vi "Fetch Measurement (More).vi"(0 "VISA resource name":refnum<visa-resource-name>, 5 "Measurement Source (1: Channel 1)":i32(ring)=1 caption="Channel (1: Channel 1)" items=["Channel 1"=1, "Channel 2"=2, "Channel 3"=3, "Channel 4"=4, "Function 1"=5, "Function 2"=6, "Function 3"=7, "Function 4"=8, "Memory 1"=9, "Memory 2"=10, "Memory 3"=11, "Memory 4"=12, "Clock"=15, "MTrend"=16, "MSpectrum"=17, "Equalized"=18, "DIG 0"=20, "DIG 1"=21, "DIG 2"=22, "DIG 3"=23, "DIG 4"=24, "DIG 5"=25, "DIG 6"=26, "DIG 7"=27, "DIG 8"=28, "DIG 9"=29, "DIG 10"=30, "DIG 11"=31, "DIG 12"=32, "DIG 13"=33, "DIG 14"=34, "DIG 15"=35], 7 "Measurement Function (0: Rise Time)":i32(ring) items=["Rise Time", "Fall Time", "Frequency", "Period", "Voltage RMS (AC)", "Voltage RMS (DC)", "Voltage RMS (AC,cycle)", "Voltage RMS (DC,cycle)", "Voltage Max", "Voltage Min", "Voltage Middle", "Voltage Vpp", "Voltage High", "Voltage Low", "Voltage Average", "Voltage Average (cycle)", "Width Negative", "Width Positive", "Duty Cycle Positive", "Amplitude", "Overshoot", "Preshoot", "Voltage Base", "Voltage Upper", "Time Max", "Time Min", "Color Grade Crossing", "Color Grade Eye Width", "Color Grade Eye Height", "Color Grade Eye Q-Factory", "Color Grade Eye Duty Cycle Distortion (Percent)", "Color Grade Eye Duty Cycle Distortion (Time)", "Color Grade Eye Jitter (PP)", "Color Grade Eye Width (RMS)", "Cycle-cycle Duty Jitter (Rising)", "Cycle-cycle Duty Jitter (Falling)", "Cycle-cycle Jitter (Rising)", "Cycle-cycle Jitter (Falling)", "Cycle-cycle - Width", "Cycle-cycle + Width", "Date Rate", "Unit Interval", "FFT Delta Frequency", "FFT Delta Magnitude", "FFT Frequency", "FFT Magnitude", "Slew Rate", "Area (Entire Display)", "Area (Single Cycle)", "Duty Cycle (Rising)", "Duty Cycle (Falling)", "Clock Recovery Rate", "Color Grade Eye Height (Measured)", "Color Grade Eye Height (Extrapolated)", "Color Grade Eye Width (Measured)", "Color Grade Eye width (Extrapolated)"], 9 "Waveform Source (1: Channel 1)":i32(ring) items=["Channel 1", "Channel 2", "Channel 3", "Channel 4", "Function 1", "Function 2", "Function 3", "Function 4", "Function 5", "Function 6", "Function 7", "Function 8", "Function 9", "Function 10", "Function 11", "Function 12", "Function 13", "Function 14", "Function 15", "Function 16", "Memory 1", "Memory 2", "Memory 3", "Memory 4", "Equalized", "MTRend", "MSPectrum"], 11 "error in (no error)":errorcluster) -> (4 "VISA resource name out":refnum<visa-resource-name>, 6 "Measurement":dbl, 15 "error out":errorcluster)   [LabVIEW 2013, in "Agilent 90000 Series.lvlib"]
doc: "Fetches the measurement result for the selected measurement.\n\nNotes:\n\n(1) You must configure the appropriate reference levels before you call this VI to take measurement.\n\n(2) You configure the low, mid, and high references either by calling the Configure Reference Levels VI.\n\n(3) This VI does not check the instrument status. Typically, you call this VI only in a sequence of calls to other low-level driver VIs. The sequence performs one operation. You use the low-level VIs to optimize one or more aspects of interaction with the instrument. If you want to check the instrument status, call the Error-Query VI at the conclusion of the sequence.\n\n(4)Duty cycle (rising) and Duty cycle (falling) have been added to the Measurement Function ring control. Data Rate and Unit Interval have their own VI which has added functionality."
uses:
  Agilent 90000 Series.lvlib
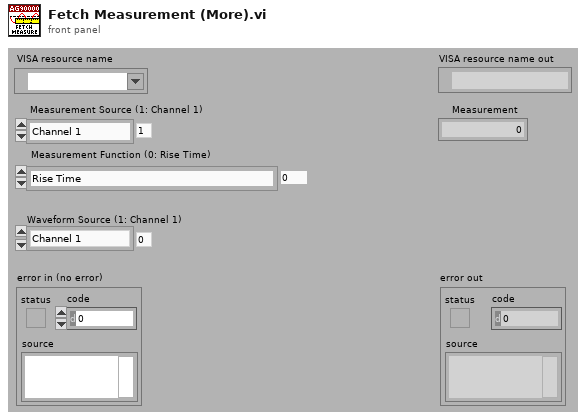
[diagram p1: front panel]
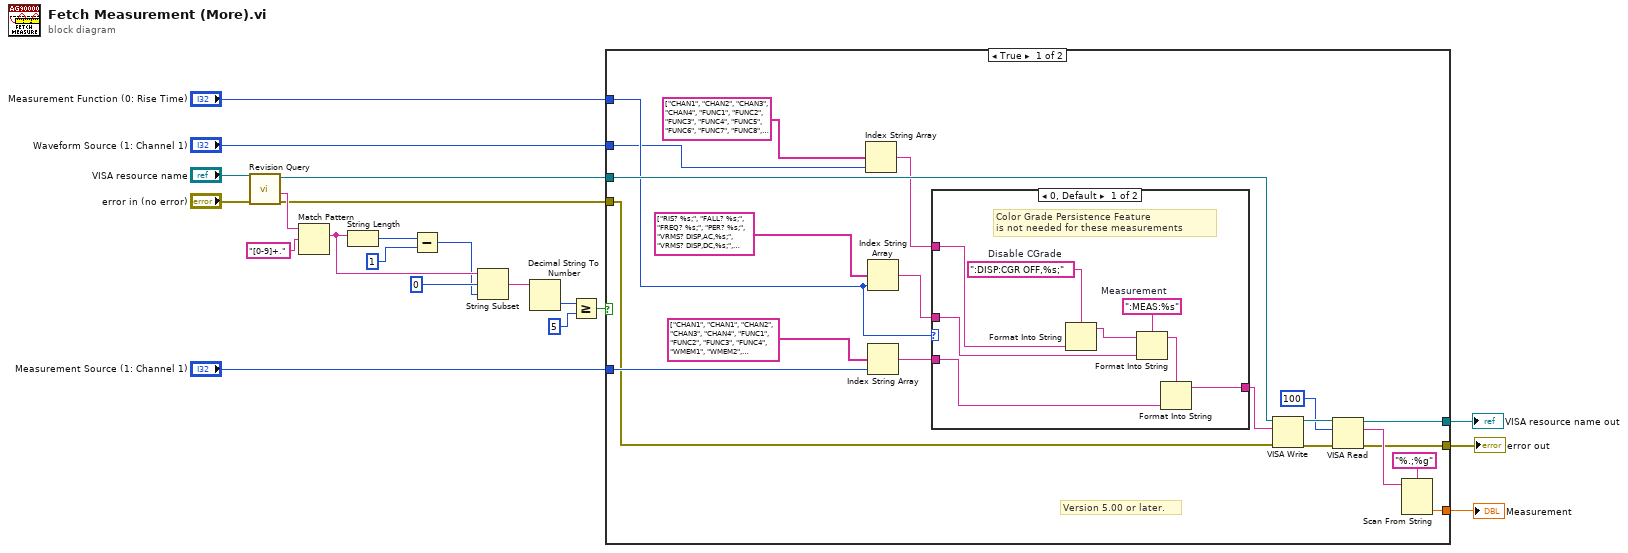
[diagram p0: block diagram]
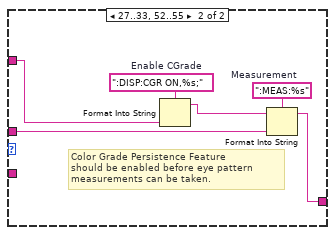
[diagram p2: hidden frame]
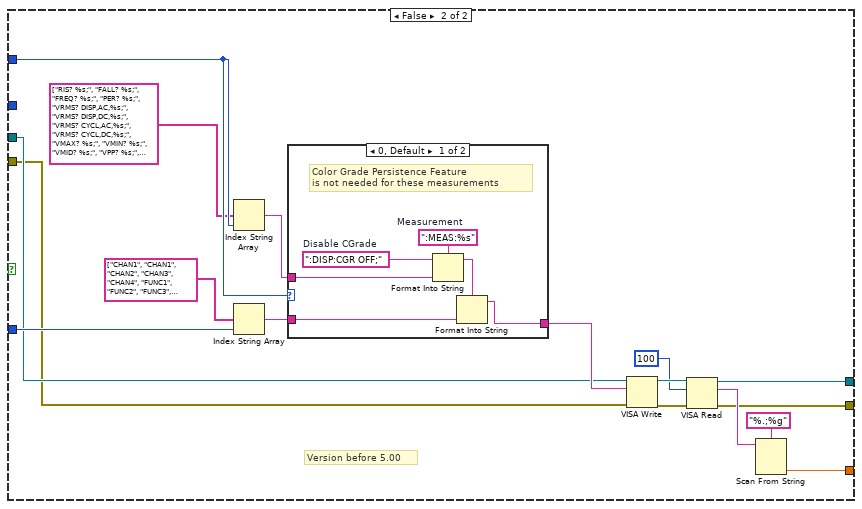
[diagram p3: hidden frame]
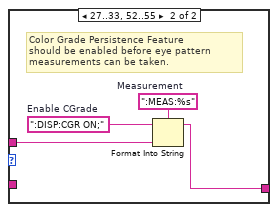
[diagram p4: hidden frame]
diagram:
  n1 = call "Revision Query.vi"("error in (no error)"="error in (no error)", "VISA resource name"="VISA resource name") -> ("error out"=w8:errorcluster, "Instrument Firmware Revision"=w10:string, "VISA resource name out"=w9:refnum<visa-resource-name>)  [unwired: 6 in, 1 out]
  n2 = Match Pattern(string=w10, regular expression="[0-9]+.") -> (match substring=w18:string)  [unwired: 1 in, 3 out]
  n3 = String Length(string=w18) -> (length=w16:i32)
  n4 = Subtract(x=w16, y=1) -> (x-y=w14:i32)
  n5 = String Subset(string=w18, offset (0)=0, length (rest)=w14) -> (substring=w13:string)
  n6 = Decimal String To Number(string=w13) -> (number=w12:i32)  [unwired: 2 in, 1 out]
  n7 = Greater Or Equal?(x=w12, y=5) -> (x >= y?=w1:bool)
  n8 = case shown="True" w1 {
    tunnel: "Measurement Function (0: Rise Time)" -> [w25 w64]
    tunnel: "Measurement Source (1: Channel 1)" -> [w33 w61]
    tunnel: w9 -> [w30 w60]
    tunnel: w8 -> [w29 w59]
    tunnel: [w28 w56] -> w3
    tunnel: [w27 w58] -> w4
    tunnel: [w26 w57] -> w2
    tunnel: "Waveform Source (1: Channel 1)" -> [w24 _]
    frame True {
      # "Version 5.00 or later."
      n9 = Index String Array(1:w24, 2:string[] ["CHAN1", "CHAN2", "CHAN3", "CHAN4", "FUNC1", "FUNC2", "FUNC3", "FUNC4", "FUNC5", "FUNC6", "FUNC7", "FUNC8", "FUNC9", "FUNC10", "FUNC11", "FUNC12", "FUNC13", "FUNC14", "FUNC15", "FUNC16", "WMEM1", "WMEM2", "WMEM3", "WMEM4", "EQU", "MTR", "MSP"] ("string array")) -> (0:w22:string)  [unwired: 1 out]
      n10 = Index String Array(1:w25, 2:string[] ["RIS? %s;", "FALL? %s;", "FREQ? %s;", "PER? %s;", "VRMS? DISP,AC,%s;", "VRMS? DISP,DC,%s;", "VRMS? CYCL,AC,%s;", "VRMS? CYCL,DC,%s;", "VMAX? %s;", "VMIN? %s;", "VMID? %s;", "VPP? %s;", "VTOP? %s;", "VLOW? %s;", "VAV? DISP,%s;", "VAV? CYCL,%s;", "NWID? %s;", "PWID? %s;", "DUTY? %s;", "VAMP? %s;", "OVER? %s;", "PRES? %s;", "VBAS? %s;", "VUPP? %s;", "TMAX? %s;", "TMIN? %s;", "CGR:CROS?;", "CGR:EWID?;", "CGR:EHE?;", "CGR:QFAC?;", "CGR:DCD? PERC;", "CGR:DCD? TIME;", "CGR:JITT? PP;", "CGR:JITT? RMS;", "CTCD? %s,RIS;", "CTCD? %s,FALL;", "CTCJ? %s,RIS;", "CTCJ? %s,FALL;", "CTCN? %s;", "CTCP? %s;", "DAT? %s;", "UNIT? %s;", "FFT:DFR? %s;", "FFT:DMAG? %s;", "FFT:FREQ? %s;", "FFT:MAGN? %s;", "SLEW? %s;", "AREA? DISP,%s;", "AREA? CYCL,%s;", "DUTY? %s,RIS;", "DUTY? %s,FALL;", "CDRRATE? %s;", "CGR:EHE? MEAS;", "CGR:EHE? EXTRapolated;", "CGR:EWID? MEAS;", "CGR:EWID? EXTRapolated;"]) -> (0:w34:string)  [unwired: 1 out]
      n11 = Index String Array(1:w33, 2:string[] ["CHAN1", "CHAN1", "CHAN2", "CHAN3", "CHAN4", "FUNC1", "FUNC2", "FUNC3", "FUNC4", "WMEM1", "WMEM2", "WMEM3", "WMEM4", "AUX", "LINE", "CLOC", "MTR", "MSP", "EQU", "NONE", "DIG0", "DIG1", "DIG2", "DIG3", "DIG4", "DIG5", "DIG6", "DIG7", "DIG8", "DIG9", "DIG10", "DIG11", "DIG12", "DIG13", "DIG14", "DIG15", "", "", "", "", "", "POD1", "POD2", "", "", "", "", "", "", "", "", "BUS1", "BUS2", "BUS3", "BUS4", "", "", "", "", "", "", "DIFF1", "DIFF2", "", "", "", "", "", "", "", "", "COMM3", "COMM4"]) -> (0:w32:string)  [unwired: 1 out]
      n12 = case shown="0, Default" w25 {
        tunnel: w34 -> [w47 w53]
        tunnel: w32 -> [w46 _]
        tunnel: [w44 w54] -> w31
        tunnel: w22 -> [w45 w51]
        frame 0, Default {
          w43 = ":DISP:CGR OFF,%s;"  # Disable CGrade
          w49 = ":MEAS:%s"  # Measurement
          # "Color Grade Persistence Feature\nis not needed for these measurements"
          n13 = Format Into String(format string=w43, w45) -> (resulting string=w42:string)  [unwired: 2 in, 1 out]
          n14 = Format Into String(format string=w49, initial string=w42, w47) -> (resulting string=w48:string)  [unwired: 1 in, 1 out]
          n15 = Format Into String(format string=w48, w46) -> (resulting string=w44:string)  [unwired: 2 in, 1 out]
        }
        frame 27..33, 52..55 {
          w52 = ":DISP:CGR ON,%s;"  # Enable CGrade
          w55 = ":MEAS:%s"  # Measurement
          # "Color Grade Persistence Feature\nshould be enabled before eye pattern\nmeasurements can be taken."
          n16 = Format Into String(format string=w52, w51) -> (resulting string=w50:string)  [unwired: 2 in, 1 out]
          n17 = Format Into String(format string=w55, initial string=w50, w53) -> (resulting string=w54:string)  [unwired: 1 in, 1 out]
        }
      }
      n18 = VISA Write(VISA resource name=w30, write buffer=w31, error in (no error)=w29) -> (VISA resource name out=w41:refnum<visa-resource-name>, error out=w40:errorcluster)  [unwired: 1 out]
      n19 = VISA Read(VISA resource name=w41, byte count=u32 100, error in (no error)=w40) -> (VISA resource name out=w28:refnum<visa-resource-name>, read buffer=w38:string, error out=w27:errorcluster)  [unwired: 1 out]
      n20 = Scan From String(format string="%.;%g", input string=w38) -> (output 1=w26:dbl)  [unwired: 2 in, 4 out]
    }
    frame False {
      # "Version before 5.00"
      n21 = Index String Array(1:w64, 2:string[] ["RIS? %s;", "FALL? %s;", "FREQ? %s;", "PER? %s;", "VRMS? DISP,AC,%s;", "VRMS? DISP,DC,%s;", "VRMS? CYCL,AC,%s;", "VRMS? CYCL,DC,%s;", "VMAX? %s;", "VMIN? %s;", "VMID? %s;", "VPP? %s;", "VTOP? %s;", "VLOW? %s;", "VAV? DISP,%s;", "VAV? CYCL,%s;", "NWID? %s;", "PWID? %s;", "DUTY? %s;", "VAMP? %s;", "OVER? %s;", "PRES? %s;", "VBAS? %s;", "VUPP? %s;", "TMAX? %s;", "TMIN? %s;", "CGR:CROS?;", "CGR:EWID?;", "CGR:EHE?;", "CGR:QFAC?;", "CGR:DCD? PERC;", "CGR:DCD? TIME;", "CGR:JITT? PP;", "CGR:JITT? RMS;", "CTCD? %s,RIS;", "CTCD? %s,FALL;", "CTCJ? %s,RIS;", "CTCJ? %s,FALL;", "CTCN? %s;", "CTCP? %s;", "DAT? %s;", "UNIT? %s;", "FFT:DFR? %s;", "FFT:DMAG? %s;", "FFT:FREQ? %s;", "FFT:MAGN? %s;", "SLEW? %s;", "AREA? DISP,%s;", "AREA? CYCL,%s;", "DUTY? %s,RIS;", "DUTY? %s,FALL;", "CDRRATE? %s;", "CGR:EHE? MEAS;", "CGR:EHE? EXTRapolated;", "CGR:EWID? MEAS;", "CGR:EWID? EXTRapolated;"]) -> (0:w72:string)  [unwired: 1 out]
      n22 = Index String Array(1:w61, 2:string[] ["CHAN1", "CHAN1", "CHAN2", "CHAN3", "CHAN4", "FUNC1", "FUNC2", "FUNC3", "FUNC4", "WMEM1", "WMEM2", "WMEM3", "WMEM4", "AUX", "LINE", "CLOC", "MTR", "MSP", "EQU", "NONE", "DIG0", "DIG1", "DIG2", "DIG3", "DIG4", "DIG5", "DIG6", "DIG7", "DIG8", "DIG9", "DIG10", "DIG11", "DIG12", "DIG13", "DIG14", "DIG15", "", "", "", "", "", "POD1", "POD2", "", "", "", "", "", "", "", "", "BUS1", "BUS2", "BUS3", "BUS4", "", "", "", "", "", "", "DIFF1", "DIFF2", "", "", "", "", "", "", "", "", "COMM3", "COMM4"]) -> (0:w66:string)  [unwired: 1 out]
      n23 = case shown="0, Default" w64 {
        tunnel: w72 -> [w76 w81]
        tunnel: w66 -> [w74 _]
        tunnel: [w73 w79] -> w65
        frame 0, Default {
          w78 = ":DISP:CGR OFF;"  # Disable CGrade
          w77 = ":MEAS:%s"  # Measurement
          # "Color Grade Persistence Feature\nis not needed for these measurements"
          n24 = Format Into String(format string=w77, initial string=w78, w76) -> (resulting string=w75:string)  [unwired: 1 in, 1 out]
          n25 = Format Into String(format string=w75, w74) -> (resulting string=w73:string)  [unwired: 2 in, 1 out]
        }
        frame 27..33, 52..55 {
          w80 = ":DISP:CGR ON;"  # Enable CGrade
          w82 = ":MEAS:%s"  # Measurement
          # "Color Grade Persistence Feature\nshould be enabled before eye pattern\nmeasurements can be taken."
          n26 = Format Into String(format string=w82, initial string=w80, w81) -> (resulting string=w79:string)  [unwired: 1 in, 1 out]
        }
      }
      n27 = VISA Write(VISA resource name=w60, write buffer=w65, error in (no error)=w59) -> (VISA resource name out=w71:refnum<visa-resource-name>, error out=w70:errorcluster)  [unwired: 1 out]
      n28 = VISA Read(VISA resource name=w71, byte count=u32 100, error in (no error)=w70) -> (VISA resource name out=w56:refnum<visa-resource-name>, read buffer=w68:string, error out=w58:errorcluster)  [unwired: 1 out]
      n29 = Scan From String(format string="%.;%g", input string=w68) -> (output 1=w57:dbl)  [unwired: 2 in, 4 out]
    }
  }
  "error out" <- w4
  "VISA resource name out" <- w3
  "Measurement" <- w2
